vi "Autonomous Independent.vi"   [LabVIEW 2016]
doc: "This VI is called when autonomous begins, and will automatically be terminated when autonomous ends. You can carry out timed or sensor driven robot movement independently without needing to return to the caller."
uses:
  <vilib>/Rock Robotics/Network Tables/NT Read String.vi
  Robot Global Data.vi
panel:
  # "Be sure to right-click and choose Data Operations>>Make Current Value default if you want to save the array values with the VI"
types:
  T1 = typedef "WPI_MotorControlDeviceRef.ctl" = cluster{"DeviceStatus":errorcluster, "Type":T2, "PWM":cluster{"PWM Channel":T3, "DeadBand":T4}, "CAN":cluster{"Device Number":u8, "SetOutput VI Ref":variant, "GetOutput VI Ref":variant, "Enable VI Ref":variant, "Disable VI Ref":variant, "Data":variant}, "Invert":bool}
  T2 = typedef "WPI_MotorControlType.ctl" = enum16{"PWM", "CAN"}
  T3 = typedef "FPGA_DIOPWMChannel.ctl" = enum8{"PWM 0", "PWM 1", "PWM 2", "PWM 3", "PWM 4", "PWM 5", "PWM 6", "PWM 7", "PWM 8", "PWM 9", "PWM MXP 0", "PWM MXP 1", "PWM MXP 2", "PWM MXP 3", "PWM MXP 4", "PWM MXP 5", "PWM MXP 6", "PWM MXP 7", "PWM MXP 8", "PWM MXP 9", "Invalid"}
  T4 = typedef "WPI_PWMDeadband.ctl" = cluster{"Name":string, "maxPositivePwm":i32, "minPositivePwm":i32, "centerPwm":i32, "maxNegativePwm":i32, "minNegativePwm":i32, "angularRange":u16}
  T5 = typedef "WPI_CANTalonSRX_GlobalStatus.ctl" = cluster{"Applied Throttle":dbl, "Module Enabled":bool, "CAN Error":errorcluster, "Closed Loop Error":dbl, "Forward Limit Switch Closed":bool, "Reverse Limit Switch Closed":bool, "Sensor Position":dbl, "Sensor Velocity":dbl, "Current":dbl, "Sticky Fault - Over Temp":bool, "Sticky Fault - Under Voltage":bool, "Sticky Fault - Forward Limit":bool, "Sticky Fault - Reverse Limit":bool, "Sticky Fault - Forward Soft Limit":bool, "Sticky Fault - Reverse Soft Limit":bool, "Brake is Enabled":bool, "Encoder Position":dbl, "Encoder Velocity":dbl, "Encoder Index Count":dbl, "Encoder A Pin State":bool, "Encoder B Pin State":bool, "Encoder Index Pin State":bool, "Analog In":dbl, "Analog In Velocity":dbl, "Temperature (C)":dbl, "Battery Voltage":dbl, "Control 5 Is Supported":bool, "Current Profile Slot Select":dbl, "Pos Div 8":bool, "Vel Div 4":bool, "Pulse Width Position":i32, "Pulse Width Velocity":i32, "Pulse Width Rise To Rise (us)":i32, "Pulse Width Rise To Fall (us)":i32, "Mot Prof Active Is Under Run":bool, "Mot Prof Active Has Under Run":bool, "Mot Prof Active Is Last":bool, "Mot Prof Active Velocity Only":bool, "Mot Prof Active Is Valid":bool, "Mot Prof Buffer Is Full":bool, "Mot Prof Active Profile Slot Select":i32, "Mot Prof NextID":i32, "Mot Prof Count":i32, "Mot Prof Active Velocity":dbl, "Mot Prof Active Position":dbl, "Mot Prof Output Enable":i32}
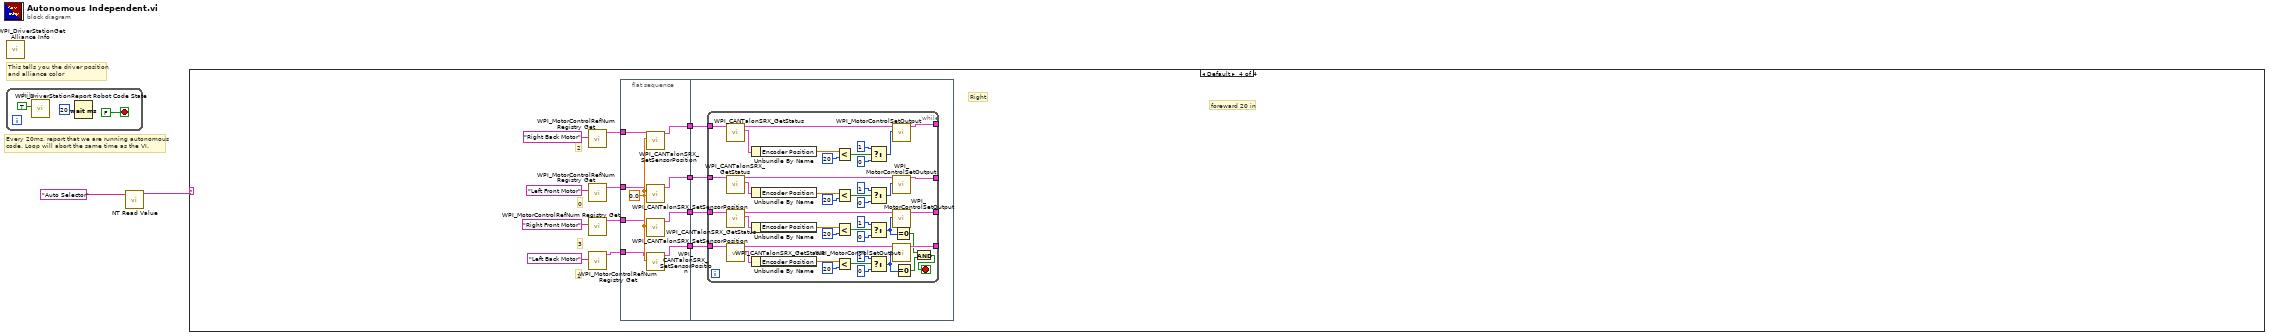
[diagram p0: block diagram]
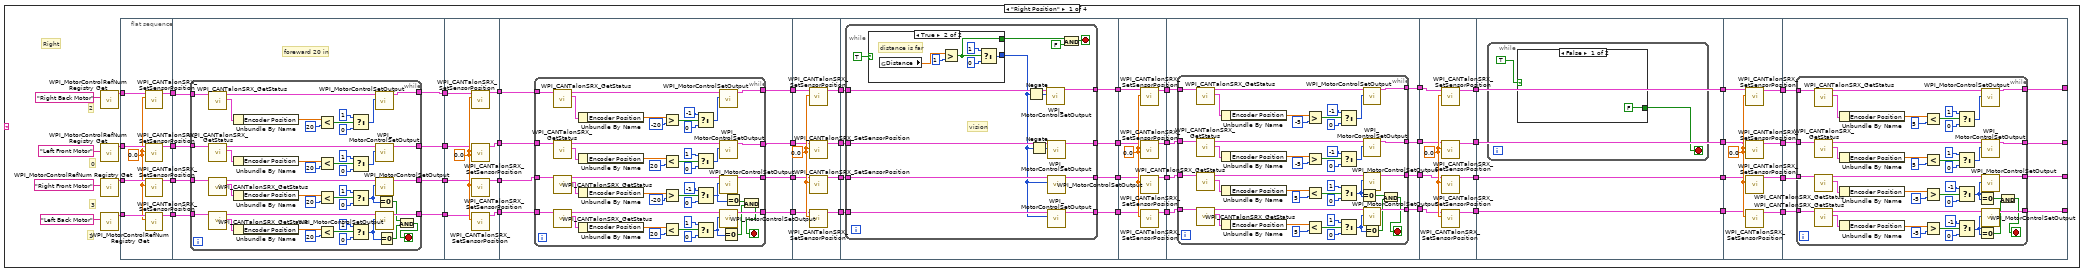
[diagram p2: hidden frame]
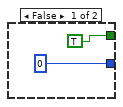
[diagram p3: hidden frame]
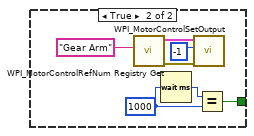
[diagram p4: hidden frame]
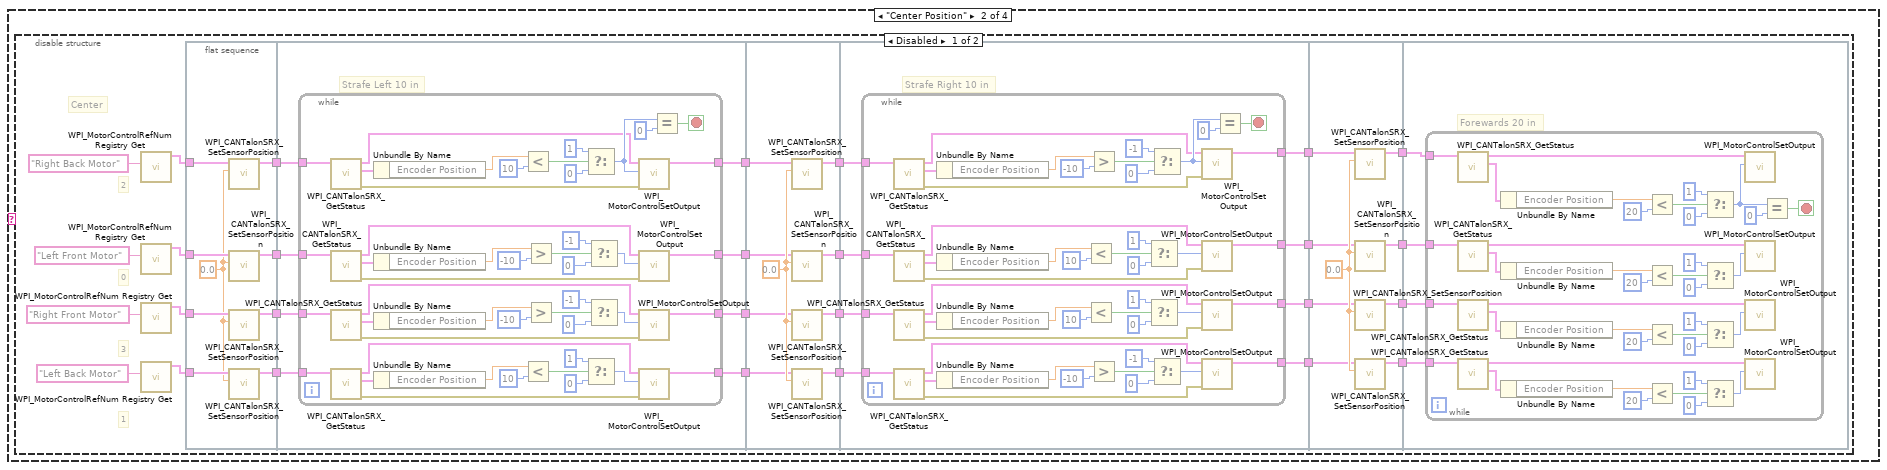
[diagram p5: hidden frame]
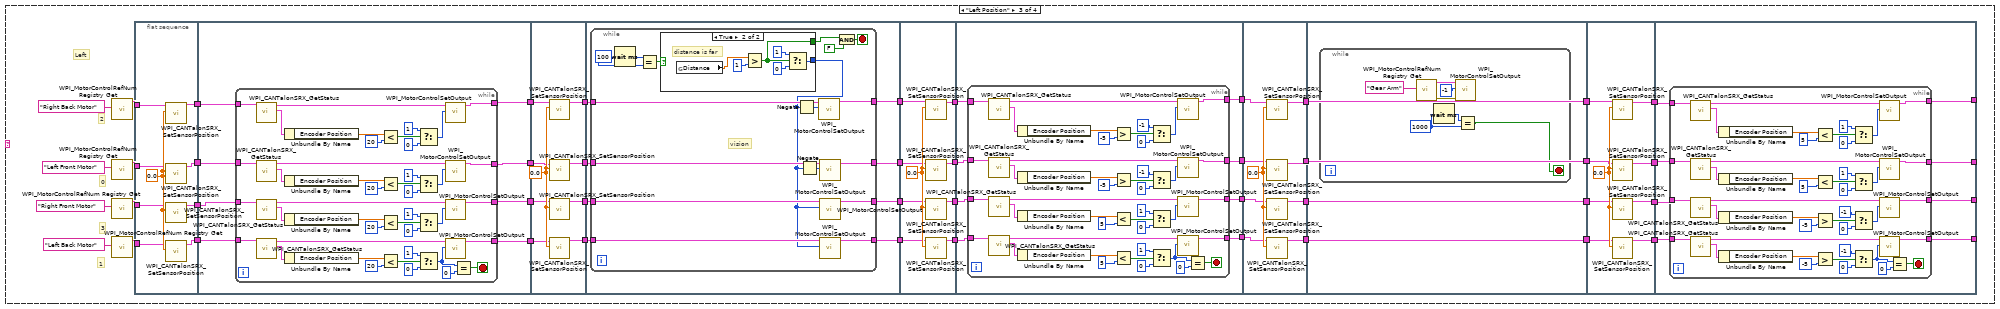
[diagram p7: hidden frame]
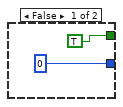
[diagram p8: hidden frame]
diagram:
  # "Every 20ms, report that we are running autonomous\ncode. Loop will abort the same time as the VI."
  # "This tells you the driver position\nand alliance color"
  n1 = call <vilib>:"WPI_DriverStationGet Alliance Info.vi"() -> ()  [unwired: 12 out]
  n2 = while {
    stop <- FALSE stop-if-true
    n3 = call <vilib>:"WPI_DriverStationReport Robot Code State.vi"("Autonomous"=TRUE) -> ()  [unwired: 10 in, 1 out]
    n4 = Wait (ms)(milliseconds to wait=u32 20) -> ()  [unwired: 1 out]
  }
  n5 = call-poly <vilib>:"NT Read Value.vi"("Name"="Auto Selector") -> ("String"=w1:string)  [unwired: 9 in, 1 out]
  n6 = case shown="Default" w1 {
    frame "Right Position" {
      # "Right"
      # "3"
      # "2"
      # "1"
      # "0"
      n7 = call <vilib>:"WPI_MotorControlRefNum Registry Get.vi"("refnum name"="Right Back Motor") -> ("MotorControlDevRef"=w42:T1)  [unwired: 9 in, 1 out]
      n8 = call <vilib>:"WPI_MotorControlRefNum Registry Get.vi"("refnum name"="Left Front Motor") -> ("MotorControlDevRef"=w43:T1)  [unwired: 9 in, 1 out]
      n9 = call <vilib>:"WPI_MotorControlRefNum Registry Get.vi"("refnum name"="Right Front Motor") -> ("MotorControlDevRef"=w44:T1)  [unwired: 9 in, 1 out]
      n10 = call <vilib>:"WPI_MotorControlRefNum Registry Get.vi"("refnum name"="Left Back Motor") -> ("MotorControlDevRef"=w45:T1)  [unwired: 9 in, 1 out]
      n11 = flat-sequence {
        tunnel: w45 -> [w65]
        tunnel: [w63] -> w57
        tunnel: w44 -> [w64]
        tunnel: w43 -> [w61]
        tunnel: [w59] -> w56
        tunnel: w42 -> [w60]
        tunnel: [w66] -> w55
        tunnel: [w62] -> w54
        tunnel: w57 -> [w71]
        tunnel: w56 -> [w73]
        tunnel: [w69] -> w53
        tunnel: [w68] -> w52
        tunnel: [w74] -> w51
        tunnel: w55 -> [w70]
        tunnel: w54 -> [w72]
        tunnel: [w67] -> w50
        tunnel: w53 -> [w122]
        tunnel: w52 -> [w123]
        tunnel: w51 -> [w125]
        tunnel: w50 -> [w124]
        tunnel: [w121] -> w37
        tunnel: [w120] -> w36
        tunnel: [w119] -> w35
        tunnel: [w118] -> w34
        tunnel: [w134] -> w41
        tunnel: [w133] -> w40
        tunnel: [w132] -> w39
        tunnel: [w131] -> w38
        tunnel: w37 -> [w130]
        tunnel: w36 -> [w129]
        tunnel: w35 -> [w128]
        tunnel: w34 -> [w127]
        tunnel: w41 -> [w185]
        tunnel: w40 -> [w184]
        tunnel: w39 -> [w183]
        tunnel: w38 -> [w182]
        tunnel: [w181] -> w33
        tunnel: [w180] -> w32
        tunnel: [w179] -> w31
        tunnel: [w178] -> w30
        tunnel: w33 -> [w194]
        tunnel: w32 -> [w193]
        tunnel: w31 -> [w192]
        tunnel: w30 -> [w191]
        tunnel: [w190] -> w29
        tunnel: [w189] -> w28
        tunnel: [w188] -> w27
        tunnel: [w187] -> w26
        tunnel: w29 -> [w225]
        tunnel: w28 -> [w224]
        tunnel: w27 -> [w223]
        tunnel: w26 -> [w222]
        tunnel: [w221] -> w25
        tunnel: [w220] -> w24
        tunnel: [w219] -> w23
        tunnel: [w218] -> w22
        tunnel: w25 -> [w231]
        tunnel: w24 -> [w232]
        tunnel: w23 -> [w233]
        tunnel: w22 -> [w234]
        tunnel: [w230] -> w21
        tunnel: [w229] -> w20
        tunnel: [w228] -> w19
        tunnel: [w227] -> w18
        tunnel: w21 -> [w285]
        tunnel: w20 -> [w283]
        tunnel: w19 -> [w281]
        tunnel: w18 -> [w279]
        tunnel: [w284] -> w17
        tunnel: [w282] -> w16
        tunnel: [w280] -> w15
        tunnel: [w278] -> w14
        tunnel: w17 -> [w290]
        tunnel: w16 -> [w289]
        tunnel: w15 -> [w288]
        tunnel: w14 -> [w287]
        tunnel: [w290] -> w13
        tunnel: [w289] -> w12
        tunnel: [w288] -> w11
        tunnel: [w287] -> w10
        tunnel: w13 -> [w308]
        tunnel: w12 -> [w307]
        tunnel: w11 -> [w306]
        tunnel: w10 -> [w305]
        tunnel: [w304] -> w9
        tunnel: [w303] -> w8
        tunnel: [w302] -> w7
        tunnel: [w301] -> w6
        tunnel: w9 -> [w314]
        tunnel: w8 -> [w315]
        tunnel: w7 -> [w316]
        tunnel: w6 -> [w317]
        tunnel: [w313] -> _
        tunnel: [w312] -> _
        tunnel: [w311] -> _
        tunnel: [w310] -> _
        frame #0 {
          w58 = 0.0
          n12 = call <vilib>:"WPI_CANTalonSRX_SetSensorPosition.vi"("New Sensor Position"=w58, "CAN Talon SRX Ref"=w60) -> ("CAN Talon SRX Ref"=w59:T1)  [unwired: 8 in, 1 out]
          n13 = call <vilib>:"WPI_CANTalonSRX_SetSensorPosition.vi"("New Sensor Position"=w58, "CAN Talon SRX Ref"=w61) -> ("CAN Talon SRX Ref"=w62:T1)  [unwired: 8 in, 1 out]
          n14 = call <vilib>:"WPI_CANTalonSRX_SetSensorPosition.vi"("New Sensor Position"=w58, "CAN Talon SRX Ref"=w64) -> ("CAN Talon SRX Ref"=w63:T1)  [unwired: 8 in, 1 out]
          n15 = call <vilib>:"WPI_CANTalonSRX_SetSensorPosition.vi"("New Sensor Position"=w58, "CAN Talon SRX Ref"=w65) -> ("CAN Talon SRX Ref"=w66:T1)  [unwired: 8 in, 1 out]
        }
        frame #1 {
          # "foreward 20 in"
          n16 = while {
            tunnel: w73 -> [w88]
            tunnel: w72 -> [w87]
            tunnel: w71 -> [w86]
            tunnel: w70 -> [w85]
            tunnel: [w83] -> w74
            tunnel: [w82] -> w69
            tunnel: [w81] -> w68
            tunnel: [w80] -> w67
            stop <- w75 stop-if-true
            n17 = call <vilib>:"WPI_CANTalonSRX_GetStatus.vi"("CAN Talon SRX Ref"=w88) -> ("Talon SRX Status"=w97:T5, "CAN Talon SRX Ref"=w96:T1)  [unwired: 8 in, 1 out]
            n18 = call <vilib>:"WPI_CANTalonSRX_GetStatus.vi"("CAN Talon SRX Ref"=w87) -> ("Talon SRX Status"=w100:T5, "CAN Talon SRX Ref"=w93:T1)  [unwired: 8 in, 1 out]
            n19 = call <vilib>:"WPI_CANTalonSRX_GetStatus.vi"("CAN Talon SRX Ref"=w86) -> ("Talon SRX Status"=w99:T5, "CAN Talon SRX Ref"=w95:T1)  [unwired: 8 in, 1 out]
            n20 = call <vilib>:"WPI_CANTalonSRX_GetStatus.vi"("CAN Talon SRX Ref"=w85) -> ("Talon SRX Status"=w98:T5, "CAN Talon SRX Ref"=w94:T1)  [unwired: 8 in, 1 out]
            n21 = Unbundle By Name(w97) -> ("Encoder Position"=w89:dbl)
            n22 = Unbundle By Name(w100) -> ("Encoder Position"=w92:dbl)
            n23 = Unbundle By Name(w99) -> ("Encoder Position"=w90:dbl)
            n24 = Unbundle By Name(w98) -> ("Encoder Position"=w91:dbl)
            n25 = Less?(x=w89, y=20) -> (x < y?=w103:bool)
            n26 = Less?(x=w92, y=20) -> (x < y?=w111:bool)
            n27 = Less?(x=w90, y=20) -> (x < y?=w109:bool)
            n28 = Less?(x=w91, y=20) -> (x < y?=w110:bool)
            n29 = Select(t=1, s=w103, f=0) -> (s? t:f=w101:i32)
            n30 = Select(t=1, s=w111, f=0) -> (s? t:f=w112:i32)
            n31 = Select(t=1, s=w109, f=0) -> (s? t:f=w79:i32)
            n32 = Select(t=1, s=w110, f=0) -> (s? t:f=w78:i32)
            n33 = call <vilib>:"WPI_MotorControlSetOutput.vi"("Output"=w101, "MotorControlDevRef"=w96) -> ("MotorControlDevRef"=w83:T1)  [unwired: 7 in, 2 out]
            n34 = call <vilib>:"WPI_MotorControlSetOutput.vi"("Output"=w112, "MotorControlDevRef"=w93) -> ("MotorControlDevRef"=w80:T1)  [unwired: 7 in, 2 out]
            n35 = call <vilib>:"WPI_MotorControlSetOutput.vi"("Output"=w79, "MotorControlDevRef"=w95) -> ("MotorControlDevRef"=w81:T1)  [unwired: 7 in, 2 out]
            n36 = call <vilib>:"WPI_MotorControlSetOutput.vi"("Output"=w78, "MotorControlDevRef"=w94) -> ("MotorControlDevRef"=w82:T1)  [unwired: 7 in, 2 out]
            n37 = Equal To 0?(x=w79) -> (x = 0?=w77:bool)
            n38 = Equal To 0?(x=w78) -> (x = 0?=w76:bool)
            n39 = And(x=w77, y=w76) -> (x .and. y?=w75:bool)
          }
        }
        frame #2 {
          w126 = 0.0
          n40 = call <vilib>:"WPI_CANTalonSRX_SetSensorPosition.vi"("New Sensor Position"=w126, "CAN Talon SRX Ref"=w125) -> ("CAN Talon SRX Ref"=w118:T1)  [unwired: 8 in, 1 out]
          n41 = call <vilib>:"WPI_CANTalonSRX_SetSensorPosition.vi"("New Sensor Position"=w126, "CAN Talon SRX Ref"=w124) -> ("CAN Talon SRX Ref"=w119:T1)  [unwired: 8 in, 1 out]
          n42 = call <vilib>:"WPI_CANTalonSRX_SetSensorPosition.vi"("New Sensor Position"=w126, "CAN Talon SRX Ref"=w123) -> ("CAN Talon SRX Ref"=w120:T1)  [unwired: 8 in, 1 out]
          n43 = call <vilib>:"WPI_CANTalonSRX_SetSensorPosition.vi"("New Sensor Position"=w126, "CAN Talon SRX Ref"=w122) -> ("CAN Talon SRX Ref"=w121:T1)  [unwired: 8 in, 1 out]
        }
        frame #3 {
          n44 = while {
            tunnel: w127 -> [w148]
            tunnel: w128 -> [w147]
            tunnel: w129 -> [w146]
            tunnel: w130 -> [w145]
            tunnel: [w143] -> w131
            tunnel: [w142] -> w134
            tunnel: [w141] -> w133
            tunnel: [w140] -> w132
            stop <- w135 stop-if-true
            n45 = call <vilib>:"WPI_CANTalonSRX_GetStatus.vi"("CAN Talon SRX Ref"=w148) -> ("Talon SRX Status"=w157:T5, "CAN Talon SRX Ref"=w156:T1)  [unwired: 8 in, 1 out]
            n46 = call <vilib>:"WPI_CANTalonSRX_GetStatus.vi"("CAN Talon SRX Ref"=w147) -> ("Talon SRX Status"=w160:T5, "CAN Talon SRX Ref"=w153:T1)  [unwired: 8 in, 1 out]
            n47 = call <vilib>:"WPI_CANTalonSRX_GetStatus.vi"("CAN Talon SRX Ref"=w146) -> ("Talon SRX Status"=w159:T5, "CAN Talon SRX Ref"=w155:T1)  [unwired: 8 in, 1 out]
            n48 = call <vilib>:"WPI_CANTalonSRX_GetStatus.vi"("CAN Talon SRX Ref"=w145) -> ("Talon SRX Status"=w158:T5, "CAN Talon SRX Ref"=w154:T1)  [unwired: 8 in, 1 out]
            n49 = Unbundle By Name(w157) -> ("Encoder Position"=w149:dbl)
            n50 = Unbundle By Name(w160) -> ("Encoder Position"=w152:dbl)
            n51 = Unbundle By Name(w159) -> ("Encoder Position"=w150:dbl)
            n52 = Unbundle By Name(w158) -> ("Encoder Position"=w151:dbl)
            n53 = Greater?(x=w149, y=-20) -> (0:w163:bool)
            n54 = Less?(x=w152, y=20) -> (x < y?=w171:bool)
            n55 = Greater?(x=w150, y=-20) -> (0:w169:bool)
            n56 = Less?(x=w151, y=20) -> (x < y?=w170:bool)
            n57 = Select(t=-1, s=w163, f=0) -> (s? t:f=w161:i32)
            n58 = Select(t=1, s=w171, f=0) -> (s? t:f=w172:i32)
            n59 = Select(t=-1, s=w169, f=0) -> (s? t:f=w138:i32)
            n60 = Select(t=1, s=w170, f=0) -> (s? t:f=w139:i32)
            n61 = call <vilib>:"WPI_MotorControlSetOutput.vi"("Output"=w161, "MotorControlDevRef"=w156) -> ("MotorControlDevRef"=w143:T1)  [unwired: 7 in, 2 out]
            n62 = call <vilib>:"WPI_MotorControlSetOutput.vi"("Output"=w172, "MotorControlDevRef"=w153) -> ("MotorControlDevRef"=w140:T1)  [unwired: 7 in, 2 out]
            n63 = call <vilib>:"WPI_MotorControlSetOutput.vi"("Output"=w138, "MotorControlDevRef"=w155) -> ("MotorControlDevRef"=w141:T1)  [unwired: 7 in, 2 out]
            n64 = call <vilib>:"WPI_MotorControlSetOutput.vi"("Output"=w139, "MotorControlDevRef"=w154) -> ("MotorControlDevRef"=w142:T1)  [unwired: 7 in, 2 out]
            n65 = Equal To 0?(x=w139) -> (x = 0?=w136:bool)
            n66 = Equal To 0?(x=w138) -> (x = 0?=w137:bool)
            n67 = And(x=w137, y=w136) -> (x .and. y?=w135:bool)
          }
        }
        frame #4 {
          w186 = 0.0
          n68 = call <vilib>:"WPI_CANTalonSRX_SetSensorPosition.vi"("New Sensor Position"=w186, "CAN Talon SRX Ref"=w182) -> ("CAN Talon SRX Ref"=w181:T1)  [unwired: 8 in, 1 out]
          n69 = call <vilib>:"WPI_CANTalonSRX_SetSensorPosition.vi"("New Sensor Position"=w186, "CAN Talon SRX Ref"=w183) -> ("CAN Talon SRX Ref"=w180:T1)  [unwired: 8 in, 1 out]
          n70 = call <vilib>:"WPI_CANTalonSRX_SetSensorPosition.vi"("New Sensor Position"=w186, "CAN Talon SRX Ref"=w184) -> ("CAN Talon SRX Ref"=w179:T1)  [unwired: 8 in, 1 out]
          n71 = call <vilib>:"WPI_CANTalonSRX_SetSensorPosition.vi"("New Sensor Position"=w186, "CAN Talon SRX Ref"=w185) -> ("CAN Talon SRX Ref"=w178:T1)  [unwired: 8 in, 1 out]
        }
        frame #5 {
          n72 = while {
            tunnel: w194 -> [w209]
            tunnel: w193 -> [w208]
            tunnel: w192 -> [w207]
            tunnel: w191 -> [w206]
            tunnel: [w205] -> w190
            tunnel: [w204] -> w189
            tunnel: [w203] -> w188
            tunnel: [w202] -> w187
            stop <- w198 stop-if-true
            # "vision"
            n73 = case shown="True" TRUE {
              tunnel: [0 w214] -> w201
              tunnel: [TRUE w213] -> w197
              frame False {
              }
              frame True {
                # "distance is far"
                n74 = global read "Robot Global Data.vi" "Distance"() -> (w212:dbl)
                n75 = Greater?(x=w212, y=1) -> (0:w213:bool)
                n76 = Select(t=1, s=w213, f=0) -> (s? t:f=w214:i32)
              }
            }
            n77 = Negate(x=w201) -> (-x=w200:i32)
            n78 = Negate(x=w201) -> (-x=w199:i32)
            n79 = call <vilib>:"WPI_MotorControlSetOutput.vi"("Output"=w200, "MotorControlDevRef"=w209) -> ("MotorControlDevRef"=w205:T1)  [unwired: 7 in, 2 out]
            n80 = call <vilib>:"WPI_MotorControlSetOutput.vi"("Output"=w199, "MotorControlDevRef"=w208) -> ("MotorControlDevRef"=w204:T1)  [unwired: 7 in, 2 out]
            n81 = call <vilib>:"WPI_MotorControlSetOutput.vi"("Output"=w201, "MotorControlDevRef"=w207) -> ("MotorControlDevRef"=w203:T1)  [unwired: 7 in, 2 out]
            n82 = call <vilib>:"WPI_MotorControlSetOutput.vi"("Output"=w201, "MotorControlDevRef"=w206) -> ("MotorControlDevRef"=w202:T1)  [unwired: 7 in, 2 out]
            n83 = And(x=w197, y=FALSE) -> (x .and. y?=w198:bool)
          }
        }
        frame #6 {
          w226 = 0.0
          n84 = call <vilib>:"WPI_CANTalonSRX_SetSensorPosition.vi"("New Sensor Position"=w226, "CAN Talon SRX Ref"=w225) -> ("CAN Talon SRX Ref"=w218:T1)  [unwired: 8 in, 1 out]
          n85 = call <vilib>:"WPI_CANTalonSRX_SetSensorPosition.vi"("New Sensor Position"=w226, "CAN Talon SRX Ref"=w224) -> ("CAN Talon SRX Ref"=w219:T1)  [unwired: 8 in, 1 out]
          n86 = call <vilib>:"WPI_CANTalonSRX_SetSensorPosition.vi"("New Sensor Position"=w226, "CAN Talon SRX Ref"=w223) -> ("CAN Talon SRX Ref"=w220:T1)  [unwired: 8 in, 1 out]
          n87 = call <vilib>:"WPI_CANTalonSRX_SetSensorPosition.vi"("New Sensor Position"=w226, "CAN Talon SRX Ref"=w222) -> ("CAN Talon SRX Ref"=w221:T1)  [unwired: 8 in, 1 out]
        }
        frame #7 {
          n88 = while {
            tunnel: w234 -> [w248]
            tunnel: w233 -> [w247]
            tunnel: w232 -> [w246]
            tunnel: w231 -> [w245]
            tunnel: [w243] -> w230
            tunnel: [w242] -> w227
            tunnel: [w241] -> w228
            tunnel: [w240] -> w229
            stop <- w235 stop-if-true
            n89 = call <vilib>:"WPI_CANTalonSRX_GetStatus.vi"("CAN Talon SRX Ref"=w248) -> ("Talon SRX Status"=w257:T5, "CAN Talon SRX Ref"=w256:T1)  [unwired: 8 in, 1 out]
            n90 = call <vilib>:"WPI_CANTalonSRX_GetStatus.vi"("CAN Talon SRX Ref"=w247) -> ("Talon SRX Status"=w260:T5, "CAN Talon SRX Ref"=w253:T1)  [unwired: 8 in, 1 out]
            n91 = call <vilib>:"WPI_CANTalonSRX_GetStatus.vi"("CAN Talon SRX Ref"=w246) -> ("Talon SRX Status"=w259:T5, "CAN Talon SRX Ref"=w255:T1)  [unwired: 8 in, 1 out]
            n92 = call <vilib>:"WPI_CANTalonSRX_GetStatus.vi"("CAN Talon SRX Ref"=w245) -> ("Talon SRX Status"=w258:T5, "CAN Talon SRX Ref"=w254:T1)  [unwired: 8 in, 1 out]
            n93 = Unbundle By Name(w257) -> ("Encoder Position"=w249:dbl)
            n94 = Unbundle By Name(w260) -> ("Encoder Position"=w252:dbl)
            n95 = Unbundle By Name(w259) -> ("Encoder Position"=w250:dbl)
            n96 = Unbundle By Name(w258) -> ("Encoder Position"=w251:dbl)
            n97 = Greater?(x=w249, y=-5) -> (0:w263:bool)
            n98 = Greater?(x=w252, y=-5) -> (0:w271:bool)
            n99 = Less?(x=w250, y=5) -> (x < y?=w269:bool)
            n100 = Less?(x=w251, y=5) -> (x < y?=w270:bool)
            n101 = Select(t=-1, s=w263, f=0) -> (s? t:f=w261:i32)
            n102 = Select(t=-1, s=w271, f=0) -> (s? t:f=w272:i32)
            n103 = Select(t=1, s=w269, f=0) -> (s? t:f=w239:i32)
            n104 = Select(t=1, s=w270, f=0) -> (s? t:f=w237:i32)
            n105 = Equal To 0?(x=w239) -> (x = 0?=w238:bool)
            n106 = call <vilib>:"WPI_MotorControlSetOutput.vi"("Output"=w261, "MotorControlDevRef"=w256) -> ("MotorControlDevRef"=w243:T1)  [unwired: 7 in, 2 out]
            n107 = call <vilib>:"WPI_MotorControlSetOutput.vi"("Output"=w272, "MotorControlDevRef"=w253) -> ("MotorControlDevRef"=w240:T1)  [unwired: 7 in, 2 out]
            n108 = call <vilib>:"WPI_MotorControlSetOutput.vi"("Output"=w239, "MotorControlDevRef"=w255) -> ("MotorControlDevRef"=w241:T1)  [unwired: 7 in, 2 out]
            n109 = call <vilib>:"WPI_MotorControlSetOutput.vi"("Output"=w237, "MotorControlDevRef"=w254) -> ("MotorControlDevRef"=w242:T1)  [unwired: 7 in, 2 out]
            n110 = Equal To 0?(x=w237) -> (x = 0?=w236:bool)
            n111 = And(x=w238, y=w236) -> (x .and. y?=w235:bool)
          }
        }
        frame #8 {
          w286 = 0.0
          n112 = call <vilib>:"WPI_CANTalonSRX_SetSensorPosition.vi"("New Sensor Position"=w286, "CAN Talon SRX Ref"=w285) -> ("CAN Talon SRX Ref"=w284:T1)  [unwired: 8 in, 1 out]
          n113 = call <vilib>:"WPI_CANTalonSRX_SetSensorPosition.vi"("New Sensor Position"=w286, "CAN Talon SRX Ref"=w283) -> ("CAN Talon SRX Ref"=w282:T1)  [unwired: 8 in, 1 out]
          n114 = call <vilib>:"WPI_CANTalonSRX_SetSensorPosition.vi"("New Sensor Position"=w286, "CAN Talon SRX Ref"=w281) -> ("CAN Talon SRX Ref"=w280:T1)  [unwired: 8 in, 1 out]
          n115 = call <vilib>:"WPI_CANTalonSRX_SetSensorPosition.vi"("New Sensor Position"=w286, "CAN Talon SRX Ref"=w279) -> ("CAN Talon SRX Ref"=w278:T1)  [unwired: 8 in, 1 out]
        }
        frame #9 {
          n116 = while {
            stop <- w291 stop-if-true
            n117 = case shown="False" TRUE {
              tunnel: [FALSE w294] -> w291
              frame False {
              }
              frame True {
                w295 = 1000
                n118 = call <vilib>:"WPI_MotorControlRefNum Registry Get.vi"("refnum name"="Gear Arm") -> ("error out"=w300:errorcluster, "MotorControlDevRef"=w299:T1)  [unwired: 9 in]
                n119 = Wait (ms)(milliseconds to wait=w295) -> (millisecond timer value=w296:u32)
                n120 = call <vilib>:"WPI_MotorControlSetOutput.vi"("error in (no error)"=w300, "Output"=-1, "MotorControlDevRef"=w299) -> ()  [unwired: 6 in, 3 out]
                n121 = Equal?(x=w296, y=w295) -> (x = y?=w294:bool)
              }
            }
          }
        }
        frame #10 {
          w309 = 0.0
          n122 = call <vilib>:"WPI_CANTalonSRX_SetSensorPosition.vi"("New Sensor Position"=w309, "CAN Talon SRX Ref"=w308) -> ("CAN Talon SRX Ref"=w301:T1)  [unwired: 8 in, 1 out]
          n123 = call <vilib>:"WPI_CANTalonSRX_SetSensorPosition.vi"("New Sensor Position"=w309, "CAN Talon SRX Ref"=w307) -> ("CAN Talon SRX Ref"=w302:T1)  [unwired: 8 in, 1 out]
          n124 = call <vilib>:"WPI_CANTalonSRX_SetSensorPosition.vi"("New Sensor Position"=w309, "CAN Talon SRX Ref"=w306) -> ("CAN Talon SRX Ref"=w303:T1)  [unwired: 8 in, 1 out]
          n125 = call <vilib>:"WPI_CANTalonSRX_SetSensorPosition.vi"("New Sensor Position"=w309, "CAN Talon SRX Ref"=w305) -> ("CAN Talon SRX Ref"=w304:T1)  [unwired: 8 in, 1 out]
        }
        frame #11 {
          n126 = while {
            tunnel: w317 -> [w331]
            tunnel: w316 -> [w330]
            tunnel: w315 -> [w329]
            tunnel: w314 -> [w328]
            tunnel: [w326] -> w313
            tunnel: [w325] -> w310
            tunnel: [w324] -> w311
            tunnel: [w323] -> w312
            stop <- w318 stop-if-true
            n127 = call <vilib>:"WPI_CANTalonSRX_GetStatus.vi"("CAN Talon SRX Ref"=w331) -> ("Talon SRX Status"=w340:T5, "CAN Talon SRX Ref"=w339:T1)  [unwired: 8 in, 1 out]
            n128 = call <vilib>:"WPI_CANTalonSRX_GetStatus.vi"("CAN Talon SRX Ref"=w330) -> ("Talon SRX Status"=w343:T5, "CAN Talon SRX Ref"=w336:T1)  [unwired: 8 in, 1 out]
            n129 = call <vilib>:"WPI_CANTalonSRX_GetStatus.vi"("CAN Talon SRX Ref"=w329) -> ("Talon SRX Status"=w342:T5, "CAN Talon SRX Ref"=w338:T1)  [unwired: 8 in, 1 out]
            n130 = call <vilib>:"WPI_CANTalonSRX_GetStatus.vi"("CAN Talon SRX Ref"=w328) -> ("Talon SRX Status"=w341:T5, "CAN Talon SRX Ref"=w337:T1)  [unwired: 8 in, 1 out]
            n131 = Unbundle By Name(w340) -> ("Encoder Position"=w332:dbl)
            n132 = Unbundle By Name(w343) -> ("Encoder Position"=w335:dbl)
            n133 = Unbundle By Name(w342) -> ("Encoder Position"=w333:dbl)
            n134 = Unbundle By Name(w341) -> ("Encoder Position"=w334:dbl)
            n135 = Less?(x=w332, y=5) -> (x < y?=w346:bool)
            n136 = Less?(x=w335, y=5) -> (x < y?=w354:bool)
            n137 = Greater?(x=w333, y=-5) -> (0:w352:bool)
            n138 = Greater?(x=w334, y=-5) -> (0:w353:bool)
            n139 = Select(t=1, s=w346, f=0) -> (s? t:f=w344:i32)
            n140 = Select(t=1, s=w354, f=0) -> (s? t:f=w355:i32)
            n141 = Select(t=-1, s=w352, f=0) -> (s? t:f=w321:i32)
            n142 = Select(t=-1, s=w353, f=0) -> (s? t:f=w320:i32)
            n143 = Equal To 0?(x=w321) -> (x = 0?=w322:bool)
            n144 = Equal To 0?(x=w320) -> (x = 0?=w319:bool)
            n145 = call <vilib>:"WPI_MotorControlSetOutput.vi"("Output"=w344, "MotorControlDevRef"=w339) -> ("MotorControlDevRef"=w326:T1)  [unwired: 7 in, 2 out]
            n146 = call <vilib>:"WPI_MotorControlSetOutput.vi"("Output"=w355, "MotorControlDevRef"=w336) -> ("MotorControlDevRef"=w323:T1)  [unwired: 7 in, 2 out]
            n147 = call <vilib>:"WPI_MotorControlSetOutput.vi"("Output"=w321, "MotorControlDevRef"=w338) -> ("MotorControlDevRef"=w324:T1)  [unwired: 7 in, 2 out]
            n148 = call <vilib>:"WPI_MotorControlSetOutput.vi"("Output"=w320, "MotorControlDevRef"=w337) -> ("MotorControlDevRef"=w325:T1)  [unwired: 7 in, 2 out]
            n149 = And(x=w322, y=w319) -> (x .and. y?=w318:bool)
          }
        }
      }
    }
    frame "Center Position" {
      n150 = disable-structure shown="Disabled" {
        frame Disabled {
          # "Center"
          # "3"
          # "2"
          # "1"
          # "0"
          n151 = call <vilib>:"WPI_MotorControlRefNum Registry Get.vi"("refnum name"="Right Back Motor") -> ("MotorControlDevRef"=w361:T1)  [unwired: 9 in, 1 out]
          n152 = call <vilib>:"WPI_MotorControlRefNum Registry Get.vi"("refnum name"="Left Front Motor") -> ("MotorControlDevRef"=w362:T1)  [unwired: 9 in, 1 out]
          n153 = call <vilib>:"WPI_MotorControlRefNum Registry Get.vi"("refnum name"="Right Front Motor") -> ("MotorControlDevRef"=w363:T1)  [unwired: 9 in, 1 out]
          n154 = call <vilib>:"WPI_MotorControlRefNum Registry Get.vi"("refnum name"="Left Back Motor") -> ("MotorControlDevRef"=w364:T1)  [unwired: 9 in, 1 out]
          n155 = flat-sequence {
            tunnel: w364 -> [w396]
            tunnel: [w394] -> w388
            tunnel: w363 -> [w395]
            tunnel: w362 -> [w392]
            tunnel: [w390] -> w387
            tunnel: w361 -> [w391]
            tunnel: [w397] -> w386
            tunnel: [w393] -> w385
            tunnel: w388 -> [w404]
            tunnel: w387 -> [w402]
            tunnel: [w401] -> w384
            tunnel: [w400] -> w383
            tunnel: [w399] -> w382
            tunnel: [w398] -> w381
            tunnel: w386 -> [w405]
            tunnel: w385 -> [w403]
            tunnel: [w452] -> w380
            tunnel: w384 -> [w453]
            tunnel: w383 -> [w454]
            tunnel: [w456] -> w379
            tunnel: w382 -> [w457]
            tunnel: w381 -> [w458]
            tunnel: [w459] -> w378
            tunnel: [w455] -> w377
            tunnel: w380 -> [w468]
            tunnel: w379 -> [w466]
            tunnel: [w464] -> w376
            tunnel: [w463] -> w375
            tunnel: [w462] -> w374
            tunnel: [w461] -> w373
            tunnel: w378 -> [w465]
            tunnel: w377 -> [w467]
            tunnel: [w521] -> w372
            tunnel: w376 -> [w522]
            tunnel: w375 -> [w515]
            tunnel: [w520] -> w371
            tunnel: w374 -> [w516]
            tunnel: w373 -> [w517]
            tunnel: [w519] -> w370
            tunnel: [w518] -> w369
            tunnel: w372 -> [w527]
            tunnel: w371 -> [w526]
            tunnel: w370 -> [w525]
            tunnel: w369 -> [w524]
            frame #0 {
              w389 = 0.0
              n156 = call <vilib>:"WPI_CANTalonSRX_SetSensorPosition.vi"("New Sensor Position"=w389, "CAN Talon SRX Ref"=w391) -> ("CAN Talon SRX Ref"=w390:T1)  [unwired: 8 in, 1 out]
              n157 = call <vilib>:"WPI_CANTalonSRX_SetSensorPosition.vi"("New Sensor Position"=w389, "CAN Talon SRX Ref"=w392) -> ("CAN Talon SRX Ref"=w393:T1)  [unwired: 8 in, 1 out]
              n158 = call <vilib>:"WPI_CANTalonSRX_SetSensorPosition.vi"("New Sensor Position"=w389, "CAN Talon SRX Ref"=w395) -> ("CAN Talon SRX Ref"=w394:T1)  [unwired: 8 in, 1 out]
              n159 = call <vilib>:"WPI_CANTalonSRX_SetSensorPosition.vi"("New Sensor Position"=w389, "CAN Talon SRX Ref"=w396) -> ("CAN Talon SRX Ref"=w397:T1)  [unwired: 8 in, 1 out]
            }
            frame #1 {
              # "Strafe Left 10 in"
              n160 = while {
                tunnel: w405 -> [w414]
                tunnel: w404 -> [w413]
                tunnel: w403 -> [w412]
                tunnel: w402 -> [w411]
                tunnel: [w409] -> w401
                tunnel: [w408] -> w400
                tunnel: [w407] -> w399
                tunnel: [w406] -> w398
                stop <- w410 stop-if-true
                n161 = call <vilib>:"WPI_CANTalonSRX_GetStatus.vi"("CAN Talon SRX Ref"=w411) -> ("error out"=w422:errorcluster, "Talon SRX Status"=w415:T5, "CAN Talon SRX Ref"=w423:T1)  [unwired: 8 in]
                n162 = call <vilib>:"WPI_CANTalonSRX_GetStatus.vi"("CAN Talon SRX Ref"=w412) -> ("error out"=w418:errorcluster, "Talon SRX Status"=w417:T5, "CAN Talon SRX Ref"=w419:T1)  [unwired: 8 in]
                n163 = call <vilib>:"WPI_CANTalonSRX_GetStatus.vi"("CAN Talon SRX Ref"=w413) -> ("error out"=w420:errorcluster, "Talon SRX Status"=w416:T5, "CAN Talon SRX Ref"=w421:T1)  [unwired: 8 in]
                n164 = call <vilib>:"WPI_CANTalonSRX_GetStatus.vi"("CAN Talon SRX Ref"=w414) -> ("error out"=w426:errorcluster, "Talon SRX Status"=w425:T5, "CAN Talon SRX Ref"=w427:T1)  [unwired: 8 in]
                n165 = Unbundle By Name(w415) -> ("Encoder Position"=w449:dbl)
                n166 = Unbundle By Name(w417) -> ("Encoder Position"=w451:dbl)
                n167 = Unbundle By Name(w416) -> ("Encoder Position"=w450:dbl)
                n168 = Unbundle By Name(w425) -> ("Encoder Position"=w424:dbl)
                n169 = Less?(x=w449, y=10) -> (x < y?=w435:bool)
                n170 = Less?(x=w424, y=10) -> (x < y?=w429:bool)
                n171 = Greater?(x=w451, y=-10) -> (0:w437:bool)
                n172 = Greater?(x=w450, y=-10) -> (0:w439:bool)
                n173 = Select(t=1, s=w435, f=0) -> (s? t:f=w433:i32)
                n174 = Select(t=1, s=w429, f=0) -> (s? t:f=w430:i32)
                n175 = Select(t=-1, s=w437, f=0) -> (s? t:f=w441:i32)
                n176 = Select(t=-1, s=w439, f=0) -> (s? t:f=w442:i32)
                n177 = call <vilib>:"WPI_MotorControlSetOutput.vi"("error in (no error)"=w422, "Output"=w433, "MotorControlDevRef"=w423) -> ("MotorControlDevRef"=w406:T1)  [unwired: 6 in, 2 out]
                n178 = call <vilib>:"WPI_MotorControlSetOutput.vi"("error in (no error)"=w418, "Output"=w441, "MotorControlDevRef"=w419) -> ("MotorControlDevRef"=w407:T1)  [unwired: 6 in, 2 out]
                n179 = call <vilib>:"WPI_MotorControlSetOutput.vi"("error in (no error)"=w420, "Output"=w442, "MotorControlDevRef"=w421) -> ("MotorControlDevRef"=w408:T1)  [unwired: 6 in, 2 out]
                n180 = call <vilib>:"WPI_MotorControlSetOutput.vi"("error in (no error)"=w426, "Output"=w430, "MotorControlDevRef"=w427) -> ("MotorControlDevRef"=w409:T1)  [unwired: 6 in, 2 out]
                n181 = Equal?(x=w433, y=0) -> (x = y?=w410:bool)
              }
            }
            frame #2 {
              w460 = 0.0
              n182 = call <vilib>:"WPI_CANTalonSRX_SetSensorPosition.vi"("New Sensor Position"=w460, "CAN Talon SRX Ref"=w458) -> ("CAN Talon SRX Ref"=w459:T1)  [unwired: 8 in, 1 out]
              n183 = call <vilib>:"WPI_CANTalonSRX_SetSensorPosition.vi"("New Sensor Position"=w460, "CAN Talon SRX Ref"=w457) -> ("CAN Talon SRX Ref"=w456:T1)  [unwired: 8 in, 1 out]
              n184 = call <vilib>:"WPI_CANTalonSRX_SetSensorPosition.vi"("New Sensor Position"=w460, "CAN Talon SRX Ref"=w454) -> ("CAN Talon SRX Ref"=w455:T1)  [unwired: 8 in, 1 out]
              n185 = call <vilib>:"WPI_CANTalonSRX_SetSensorPosition.vi"("New Sensor Position"=w460, "CAN Talon SRX Ref"=w453) -> ("CAN Talon SRX Ref"=w452:T1)  [unwired: 8 in, 1 out]
            }
            frame #3 {
              # "Strafe Right 10 in"
              n186 = while {
                tunnel: w468 -> [w477]
                tunnel: w467 -> [w476]
                tunnel: w465 -> [w475]
                tunnel: w466 -> [w473]
                tunnel: [w472] -> w464
                tunnel: [w471] -> w463
                tunnel: [w470] -> w462
                tunnel: [w469] -> w461
                stop <- w474 stop-if-true
                n187 = call <vilib>:"WPI_CANTalonSRX_GetStatus.vi"("CAN Talon SRX Ref"=w475) -> ("error out"=w485:errorcluster, "Talon SRX Status"=w478:T5, "CAN Talon SRX Ref"=w486:T1)  [unwired: 8 in]
                n188 = call <vilib>:"WPI_CANTalonSRX_GetStatus.vi"("CAN Talon SRX Ref"=w473) -> ("error out"=w481:errorcluster, "Talon SRX Status"=w480:T5, "CAN Talon SRX Ref"=w482:T1)  [unwired: 8 in]
                n189 = call <vilib>:"WPI_CANTalonSRX_GetStatus.vi"("CAN Talon SRX Ref"=w476) -> ("error out"=w483:errorcluster, "Talon SRX Status"=w479:T5, "CAN Talon SRX Ref"=w484:T1)  [unwired: 8 in]
                n190 = call <vilib>:"WPI_CANTalonSRX_GetStatus.vi"("CAN Talon SRX Ref"=w477) -> ("error out"=w489:errorcluster, "Talon SRX Status"=w488:T5, "CAN Talon SRX Ref"=w490:T1)  [unwired: 8 in]
                n191 = Unbundle By Name(w478) -> ("Encoder Position"=w512:dbl)
                n192 = Unbundle By Name(w480) -> ("Encoder Position"=w514:dbl)
                n193 = Unbundle By Name(w479) -> ("Encoder Position"=w513:dbl)
                n194 = Unbundle By Name(w488) -> ("Encoder Position"=w487:dbl)
                n195 = Less?(x=w514, y=10) -> (x < y?=w500:bool)
                n196 = Less?(x=w513, y=10) -> (x < y?=w502:bool)
                n197 = Greater?(x=w512, y=-10) -> (0:w498:bool)
                n198 = Greater?(x=w487, y=-10) -> (0:w492:bool)
                n199 = Select(t=1, s=w500, f=0) -> (s? t:f=w504:i32)
                n200 = Select(t=1, s=w502, f=0) -> (s? t:f=w505:i32)
                n201 = Select(t=-1, s=w498, f=0) -> (s? t:f=w496:i32)
                n202 = Select(t=-1, s=w492, f=0) -> (s? t:f=w493:i32)
                n203 = call <vilib>:"WPI_MotorControlSetOutput.vi"("error in (no error)"=w485, "Output"=w496, "MotorControlDevRef"=w486) -> ("MotorControlDevRef"=w472:T1)  [unwired: 6 in, 2 out]
                n204 = call <vilib>:"WPI_MotorControlSetOutput.vi"("error in (no error)"=w481, "Output"=w504, "MotorControlDevRef"=w482) -> ("MotorControlDevRef"=w471:T1)  [unwired: 6 in, 2 out]
                n205 = call <vilib>:"WPI_MotorControlSetOutput.vi"("error in (no error)"=w483, "Output"=w505, "MotorControlDevRef"=w484) -> ("MotorControlDevRef"=w470:T1)  [unwired: 6 in, 2 out]
                n206 = call <vilib>:"WPI_MotorControlSetOutput.vi"("error in (no error)"=w489, "Output"=w493, "MotorControlDevRef"=w490) -> ("MotorControlDevRef"=w469:T1)  [unwired: 6 in, 2 out]
                n207 = Equal?(x=w496, y=0) -> (x = y?=w474:bool)
              }
            }
            frame #4 {
              w523 = 0.0
              n208 = call <vilib>:"WPI_CANTalonSRX_SetSensorPosition.vi"("New Sensor Position"=w523, "CAN Talon SRX Ref"=w522) -> ("CAN Talon SRX Ref"=w521:T1)  [unwired: 8 in, 1 out]
              n209 = call <vilib>:"WPI_CANTalonSRX_SetSensorPosition.vi"("New Sensor Position"=w523, "CAN Talon SRX Ref"=w515) -> ("CAN Talon SRX Ref"=w520:T1)  [unwired: 8 in, 1 out]
              n210 = call <vilib>:"WPI_CANTalonSRX_SetSensorPosition.vi"("New Sensor Position"=w523, "CAN Talon SRX Ref"=w516) -> ("CAN Talon SRX Ref"=w519:T1)  [unwired: 8 in, 1 out]
              n211 = call <vilib>:"WPI_CANTalonSRX_SetSensorPosition.vi"("New Sensor Position"=w523, "CAN Talon SRX Ref"=w517) -> ("CAN Talon SRX Ref"=w518:T1)  [unwired: 8 in, 1 out]
            }
            frame #5 {
              # "Forewards 20 in"
              n212 = while {
                tunnel: w527 -> [w532]
                tunnel: w526 -> [w531]
                tunnel: w525 -> [w530]
                tunnel: w524 -> [w529]
                stop <- w545 stop-if-true
                n213 = call <vilib>:"WPI_CANTalonSRX_GetStatus.vi"("CAN Talon SRX Ref"=w532) -> ("Talon SRX Status"=w541:T5, "CAN Talon SRX Ref"=w540:T1)  [unwired: 8 in, 1 out]
                n214 = call <vilib>:"WPI_CANTalonSRX_GetStatus.vi"("CAN Talon SRX Ref"=w531) -> ("Talon SRX Status"=w544:T5, "CAN Talon SRX Ref"=w537:T1)  [unwired: 8 in, 1 out]
                n215 = call <vilib>:"WPI_CANTalonSRX_GetStatus.vi"("CAN Talon SRX Ref"=w530) -> ("Talon SRX Status"=w543:T5, "CAN Talon SRX Ref"=w539:T1)  [unwired: 8 in, 1 out]
                n216 = call <vilib>:"WPI_CANTalonSRX_GetStatus.vi"("CAN Talon SRX Ref"=w529) -> ("Talon SRX Status"=w542:T5, "CAN Talon SRX Ref"=w538:T1)  [unwired: 8 in, 1 out]
                n217 = Unbundle By Name(w541) -> ("Encoder Position"=w533:dbl)
                n218 = Unbundle By Name(w544) -> ("Encoder Position"=w536:dbl)
                n219 = Unbundle By Name(w543) -> ("Encoder Position"=w534:dbl)
                n220 = Unbundle By Name(w542) -> ("Encoder Position"=w535:dbl)
                n221 = Less?(x=w533, y=20) -> (x < y?=w549:bool)
                n222 = Less?(x=w536, y=20) -> (x < y?=w557:bool)
                n223 = Less?(x=w534, y=20) -> (x < y?=w555:bool)
                n224 = Less?(x=w535, y=20) -> (x < y?=w556:bool)
                n225 = Select(t=1, s=w549, f=0) -> (s? t:f=w546:i32)
                n226 = Select(t=1, s=w557, f=0) -> (s? t:f=w560:i32)
                n227 = Select(t=1, s=w555, f=0) -> (s? t:f=w558:i32)
                n228 = Select(t=1, s=w556, f=0) -> (s? t:f=w559:i32)
                n229 = call <vilib>:"WPI_MotorControlSetOutput.vi"("Output"=w546, "MotorControlDevRef"=w540) -> ()  [unwired: 7 in, 3 out]
                n230 = call <vilib>:"WPI_MotorControlSetOutput.vi"("Output"=w560, "MotorControlDevRef"=w537) -> ()  [unwired: 7 in, 3 out]
                n231 = call <vilib>:"WPI_MotorControlSetOutput.vi"("Output"=w558, "MotorControlDevRef"=w539) -> ()  [unwired: 7 in, 3 out]
                n232 = call <vilib>:"WPI_MotorControlSetOutput.vi"("Output"=w559, "MotorControlDevRef"=w538) -> ()  [unwired: 7 in, 3 out]
                n233 = Equal?(x=w546, y=0) -> (x = y?=w545:bool)
              }
            }
          }
        }
        frame Enabled {
        }
      }
    }
    frame "Left Position" {
      # "Left"
      # "3"
      # "2"
      # "1"
      # "0"
      n234 = call <vilib>:"WPI_MotorControlRefNum Registry Get.vi"("refnum name"="Right Back Motor") -> ("MotorControlDevRef"=w566:T1)  [unwired: 9 in, 1 out]
      n235 = call <vilib>:"WPI_MotorControlRefNum Registry Get.vi"("refnum name"="Left Front Motor") -> ("MotorControlDevRef"=w567:T1)  [unwired: 9 in, 1 out]
      n236 = call <vilib>:"WPI_MotorControlRefNum Registry Get.vi"("refnum name"="Right Front Motor") -> ("MotorControlDevRef"=w568:T1)  [unwired: 9 in, 1 out]
      n237 = call <vilib>:"WPI_MotorControlRefNum Registry Get.vi"("refnum name"="Left Back Motor") -> ("MotorControlDevRef"=w569:T1)  [unwired: 9 in, 1 out]
      n238 = flat-sequence {
        tunnel: [w617] -> w609
        tunnel: [w616] -> w608
        tunnel: [w615] -> w607
        tunnel: [w614] -> w606
        tunnel: w569 -> [w613]
        tunnel: w568 -> [w612]
        tunnel: w567 -> [w611]
        tunnel: w566 -> [w610]
        tunnel: w609 -> [w619]
        tunnel: w608 -> [w620]
        tunnel: w607 -> [w621]
        tunnel: w606 -> [w622]
        tunnel: [w626] -> w573
        tunnel: [w625] -> w572
        tunnel: [w624] -> w571
        tunnel: [w623] -> w570
        tunnel: [w676] -> w605
        tunnel: [w675] -> w604
        tunnel: [w674] -> w603
        tunnel: [w673] -> w602
        tunnel: w573 -> [w672]
        tunnel: w572 -> [w671]
        tunnel: w571 -> [w670]
        tunnel: w570 -> [w669]
        tunnel: w605 -> [w685]
        tunnel: w604 -> [w684]
        tunnel: w603 -> [w683]
        tunnel: w602 -> [w682]
        tunnel: [w681] -> w601
        tunnel: [w680] -> w600
        tunnel: [w679] -> w599
        tunnel: [w678] -> w598
        tunnel: w601 -> [w718]
        tunnel: w600 -> [w717]
        tunnel: w599 -> [w716]
        tunnel: w598 -> [w715]
        tunnel: [w714] -> w597
        tunnel: [w713] -> w596
        tunnel: [w712] -> w595
        tunnel: [w711] -> w594
        tunnel: w597 -> [w724]
        tunnel: w596 -> [w725]
        tunnel: w595 -> [w726]
        tunnel: w594 -> [w727]
        tunnel: [w723] -> w593
        tunnel: [w722] -> w592
        tunnel: [w721] -> w591
        tunnel: [w720] -> w590
        tunnel: w593 -> [w777]
        tunnel: w592 -> [w775]
        tunnel: w591 -> [w773]
        tunnel: w590 -> [w771]
        tunnel: [w776] -> w589
        tunnel: [w774] -> w588
        tunnel: [w772] -> w587
        tunnel: [w770] -> w586
        tunnel: w589 -> [w782]
        tunnel: w588 -> [w781]
        tunnel: w587 -> [w780]
        tunnel: w586 -> [w779]
        tunnel: [w782] -> w585
        tunnel: [w781] -> w584
        tunnel: [w780] -> w583
        tunnel: [w779] -> w582
        tunnel: w585 -> [w797]
        tunnel: w584 -> [w796]
        tunnel: w583 -> [w795]
        tunnel: w582 -> [w794]
        tunnel: [w793] -> w581
        tunnel: [w792] -> w580
        tunnel: [w791] -> w579
        tunnel: [w790] -> w578
        tunnel: w581 -> [w803]
        tunnel: w580 -> [w804]
        tunnel: w579 -> [w805]
        tunnel: w578 -> [w806]
        tunnel: [w802] -> _
        tunnel: [w801] -> _
        tunnel: [w800] -> _
        tunnel: [w799] -> _
        frame #0 {
          w618 = 0.0
          n239 = call <vilib>:"WPI_CANTalonSRX_SetSensorPosition.vi"("New Sensor Position"=w618, "CAN Talon SRX Ref"=w610) -> ("CAN Talon SRX Ref"=w614:T1)  [unwired: 8 in, 1 out]
          n240 = call <vilib>:"WPI_CANTalonSRX_SetSensorPosition.vi"("New Sensor Position"=w618, "CAN Talon SRX Ref"=w611) -> ("CAN Talon SRX Ref"=w615:T1)  [unwired: 8 in, 1 out]
          n241 = call <vilib>:"WPI_CANTalonSRX_SetSensorPosition.vi"("New Sensor Position"=w618, "CAN Talon SRX Ref"=w612) -> ("CAN Talon SRX Ref"=w616:T1)  [unwired: 8 in, 1 out]
          n242 = call <vilib>:"WPI_CANTalonSRX_SetSensorPosition.vi"("New Sensor Position"=w618, "CAN Talon SRX Ref"=w613) -> ("CAN Talon SRX Ref"=w617:T1)  [unwired: 8 in, 1 out]
        }
        frame #1 {
          n243 = while {
            tunnel: [w635] -> w623
            tunnel: [w634] -> w626
            tunnel: [w633] -> w625
            tunnel: [w632] -> w624
            tunnel: w622 -> [w630]
            tunnel: w621 -> [w629]
            tunnel: w620 -> [w628]
            tunnel: w619 -> [w627]
            stop <- w649 stop-if-true
            n244 = call <vilib>:"WPI_CANTalonSRX_GetStatus.vi"("CAN Talon SRX Ref"=w630) -> ("Talon SRX Status"=w645:T5, "CAN Talon SRX Ref"=w644:T1)  [unwired: 8 in, 1 out]
            n245 = call <vilib>:"WPI_CANTalonSRX_GetStatus.vi"("CAN Talon SRX Ref"=w629) -> ("Talon SRX Status"=w648:T5, "CAN Talon SRX Ref"=w641:T1)  [unwired: 8 in, 1 out]
            n246 = call <vilib>:"WPI_CANTalonSRX_GetStatus.vi"("CAN Talon SRX Ref"=w628) -> ("Talon SRX Status"=w647:T5, "CAN Talon SRX Ref"=w643:T1)  [unwired: 8 in, 1 out]
            n247 = call <vilib>:"WPI_CANTalonSRX_GetStatus.vi"("CAN Talon SRX Ref"=w627) -> ("Talon SRX Status"=w646:T5, "CAN Talon SRX Ref"=w642:T1)  [unwired: 8 in, 1 out]
            n248 = Unbundle By Name(w645) -> ("Encoder Position"=w637:dbl)
            n249 = Unbundle By Name(w648) -> ("Encoder Position"=w640:dbl)
            n250 = Unbundle By Name(w647) -> ("Encoder Position"=w638:dbl)
            n251 = Unbundle By Name(w646) -> ("Encoder Position"=w639:dbl)
            n252 = Less?(x=w637, y=20) -> (x < y?=w653:bool)
            n253 = Less?(x=w640, y=20) -> (x < y?=w661:bool)
            n254 = Less?(x=w638, y=20) -> (x < y?=w659:bool)
            n255 = Less?(x=w639, y=20) -> (x < y?=w660:bool)
            n256 = Select(t=1, s=w653, f=0) -> (s? t:f=w650:i32)
            n257 = Select(t=1, s=w661, f=0) -> (s? t:f=w663:i32)
            n258 = Select(t=1, s=w659, f=0) -> (s? t:f=w662:i32)
            n259 = Select(t=1, s=w660, f=0) -> (s? t:f=w631:i32)
            n260 = call <vilib>:"WPI_MotorControlSetOutput.vi"("Output"=w650, "MotorControlDevRef"=w644) -> ("MotorControlDevRef"=w635:T1)  [unwired: 7 in, 2 out]
            n261 = call <vilib>:"WPI_MotorControlSetOutput.vi"("Output"=w663, "MotorControlDevRef"=w641) -> ("MotorControlDevRef"=w632:T1)  [unwired: 7 in, 2 out]
            n262 = call <vilib>:"WPI_MotorControlSetOutput.vi"("Output"=w662, "MotorControlDevRef"=w643) -> ("MotorControlDevRef"=w633:T1)  [unwired: 7 in, 2 out]
            n263 = call <vilib>:"WPI_MotorControlSetOutput.vi"("Output"=w631, "MotorControlDevRef"=w642) -> ("MotorControlDevRef"=w634:T1)  [unwired: 7 in, 2 out]
            n264 = Equal?(x=w631, y=0) -> (x = y?=w649:bool)
          }
        }
        frame #2 {
          w677 = 0.0
          n265 = call <vilib>:"WPI_CANTalonSRX_SetSensorPosition.vi"("New Sensor Position"=w677, "CAN Talon SRX Ref"=w669) -> ("CAN Talon SRX Ref"=w676:T1)  [unwired: 8 in, 1 out]
          n266 = call <vilib>:"WPI_CANTalonSRX_SetSensorPosition.vi"("New Sensor Position"=w677, "CAN Talon SRX Ref"=w670) -> ("CAN Talon SRX Ref"=w675:T1)  [unwired: 8 in, 1 out]
          n267 = call <vilib>:"WPI_CANTalonSRX_SetSensorPosition.vi"("New Sensor Position"=w677, "CAN Talon SRX Ref"=w671) -> ("CAN Talon SRX Ref"=w674:T1)  [unwired: 8 in, 1 out]
          n268 = call <vilib>:"WPI_CANTalonSRX_SetSensorPosition.vi"("New Sensor Position"=w677, "CAN Talon SRX Ref"=w672) -> ("CAN Talon SRX Ref"=w673:T1)  [unwired: 8 in, 1 out]
        }
        frame #3 {
          n269 = while {
            tunnel: w685 -> [w699]
            tunnel: w684 -> [w698]
            tunnel: w683 -> [w697]
            tunnel: w682 -> [w696]
            tunnel: [w695] -> w681
            tunnel: [w694] -> w680
            tunnel: [w693] -> w679
            tunnel: [w692] -> w678
            stop <- w688 stop-if-true
            w701 = 100
            # "vision"
            n270 = Wait (ms)(milliseconds to wait=w701) -> (millisecond timer value=w702:u32)
            n271 = Equal?(x=w702, y=w701) -> (x = y?=w700:bool)
            n272 = case shown="True" w700 {
              tunnel: [0 w707] -> w691
              tunnel: [TRUE w706] -> w687
              frame False {
              }
              frame True {
                # "distance is far"
                n273 = global read "Robot Global Data.vi" "Distance"() -> (w705:dbl)
                n274 = Greater?(x=w705, y=1) -> (0:w706:bool)
                n275 = Select(t=1, s=w706, f=0) -> (s? t:f=w707:i32)
              }
            }
            n276 = Negate(x=w691) -> (-x=w690:i32)
            n277 = Negate(x=w691) -> (-x=w689:i32)
            n278 = call <vilib>:"WPI_MotorControlSetOutput.vi"("Output"=w690, "MotorControlDevRef"=w699) -> ("MotorControlDevRef"=w695:T1)  [unwired: 7 in, 2 out]
            n279 = call <vilib>:"WPI_MotorControlSetOutput.vi"("Output"=w689, "MotorControlDevRef"=w698) -> ("MotorControlDevRef"=w694:T1)  [unwired: 7 in, 2 out]
            n280 = call <vilib>:"WPI_MotorControlSetOutput.vi"("Output"=w691, "MotorControlDevRef"=w697) -> ("MotorControlDevRef"=w693:T1)  [unwired: 7 in, 2 out]
            n281 = call <vilib>:"WPI_MotorControlSetOutput.vi"("Output"=w691, "MotorControlDevRef"=w696) -> ("MotorControlDevRef"=w692:T1)  [unwired: 7 in, 2 out]
            n282 = And(x=w687, y=FALSE) -> (x .and. y?=w688:bool)
          }
        }
        frame #4 {
          w719 = 0.0
          n283 = call <vilib>:"WPI_CANTalonSRX_SetSensorPosition.vi"("New Sensor Position"=w719, "CAN Talon SRX Ref"=w718) -> ("CAN Talon SRX Ref"=w711:T1)  [unwired: 8 in, 1 out]
          n284 = call <vilib>:"WPI_CANTalonSRX_SetSensorPosition.vi"("New Sensor Position"=w719, "CAN Talon SRX Ref"=w717) -> ("CAN Talon SRX Ref"=w712:T1)  [unwired: 8 in, 1 out]
          n285 = call <vilib>:"WPI_CANTalonSRX_SetSensorPosition.vi"("New Sensor Position"=w719, "CAN Talon SRX Ref"=w716) -> ("CAN Talon SRX Ref"=w713:T1)  [unwired: 8 in, 1 out]
          n286 = call <vilib>:"WPI_CANTalonSRX_SetSensorPosition.vi"("New Sensor Position"=w719, "CAN Talon SRX Ref"=w715) -> ("CAN Talon SRX Ref"=w714:T1)  [unwired: 8 in, 1 out]
        }
        frame #5 {
          n287 = while {
            tunnel: w727 -> [w737]
            tunnel: w726 -> [w736]
            tunnel: w725 -> [w735]
            tunnel: w724 -> [w734]
            tunnel: [w732] -> w723
            tunnel: [w731] -> w720
            tunnel: [w730] -> w721
            tunnel: [w729] -> w722
            stop <- w750 stop-if-true
            n288 = call <vilib>:"WPI_CANTalonSRX_GetStatus.vi"("CAN Talon SRX Ref"=w737) -> ("Talon SRX Status"=w746:T5, "CAN Talon SRX Ref"=w745:T1)  [unwired: 8 in, 1 out]
            n289 = call <vilib>:"WPI_CANTalonSRX_GetStatus.vi"("CAN Talon SRX Ref"=w736) -> ("Talon SRX Status"=w749:T5, "CAN Talon SRX Ref"=w742:T1)  [unwired: 8 in, 1 out]
            n290 = call <vilib>:"WPI_CANTalonSRX_GetStatus.vi"("CAN Talon SRX Ref"=w735) -> ("Talon SRX Status"=w748:T5, "CAN Talon SRX Ref"=w744:T1)  [unwired: 8 in, 1 out]
            n291 = call <vilib>:"WPI_CANTalonSRX_GetStatus.vi"("CAN Talon SRX Ref"=w734) -> ("Talon SRX Status"=w747:T5, "CAN Talon SRX Ref"=w743:T1)  [unwired: 8 in, 1 out]
            n292 = Unbundle By Name(w746) -> ("Encoder Position"=w738:dbl)
            n293 = Unbundle By Name(w749) -> ("Encoder Position"=w741:dbl)
            n294 = Unbundle By Name(w748) -> ("Encoder Position"=w739:dbl)
            n295 = Unbundle By Name(w747) -> ("Encoder Position"=w740:dbl)
            n296 = Greater?(x=w738, y=-5) -> (0:w754:bool)
            n297 = Greater?(x=w741, y=-5) -> (0:w762:bool)
            n298 = Less?(x=w739, y=5) -> (x < y?=w760:bool)
            n299 = Less?(x=w740, y=5) -> (x < y?=w761:bool)
            n300 = Select(t=-1, s=w754, f=0) -> (s? t:f=w751:i32)
            n301 = Select(t=-1, s=w762, f=0) -> (s? t:f=w764:i32)
            n302 = Select(t=1, s=w760, f=0) -> (s? t:f=w763:i32)
            n303 = Select(t=1, s=w761, f=0) -> (s? t:f=w728:i32)
            n304 = call <vilib>:"WPI_MotorControlSetOutput.vi"("Output"=w751, "MotorControlDevRef"=w745) -> ("MotorControlDevRef"=w732:T1)  [unwired: 7 in, 2 out]
            n305 = call <vilib>:"WPI_MotorControlSetOutput.vi"("Output"=w764, "MotorControlDevRef"=w742) -> ("MotorControlDevRef"=w729:T1)  [unwired: 7 in, 2 out]
            n306 = call <vilib>:"WPI_MotorControlSetOutput.vi"("Output"=w763, "MotorControlDevRef"=w744) -> ("MotorControlDevRef"=w730:T1)  [unwired: 7 in, 2 out]
            n307 = call <vilib>:"WPI_MotorControlSetOutput.vi"("Output"=w728, "MotorControlDevRef"=w743) -> ("MotorControlDevRef"=w731:T1)  [unwired: 7 in, 2 out]
            n308 = Equal?(x=w728, y=0) -> (x = y?=w750:bool)
          }
        }
        frame #6 {
          w778 = 0.0
          n309 = call <vilib>:"WPI_CANTalonSRX_SetSensorPosition.vi"("New Sensor Position"=w778, "CAN Talon SRX Ref"=w777) -> ("CAN Talon SRX Ref"=w776:T1)  [unwired: 8 in, 1 out]
          n310 = call <vilib>:"WPI_CANTalonSRX_SetSensorPosition.vi"("New Sensor Position"=w778, "CAN Talon SRX Ref"=w775) -> ("CAN Talon SRX Ref"=w774:T1)  [unwired: 8 in, 1 out]
          n311 = call <vilib>:"WPI_CANTalonSRX_SetSensorPosition.vi"("New Sensor Position"=w778, "CAN Talon SRX Ref"=w773) -> ("CAN Talon SRX Ref"=w772:T1)  [unwired: 8 in, 1 out]
          n312 = call <vilib>:"WPI_CANTalonSRX_SetSensorPosition.vi"("New Sensor Position"=w778, "CAN Talon SRX Ref"=w771) -> ("CAN Talon SRX Ref"=w770:T1)  [unwired: 8 in, 1 out]
        }
        frame #7 {
          n313 = while {
            stop <- w783 stop-if-true
            w784 = 1000
            n314 = call <vilib>:"WPI_MotorControlRefNum Registry Get.vi"("refnum name"="Gear Arm") -> ("error out"=w789:errorcluster, "MotorControlDevRef"=w788:T1)  [unwired: 9 in]
            n315 = Wait (ms)(milliseconds to wait=w784) -> (millisecond timer value=w785:u32)
            n316 = call <vilib>:"WPI_MotorControlSetOutput.vi"("error in (no error)"=w789, "Output"=-1, "MotorControlDevRef"=w788) -> ()  [unwired: 6 in, 3 out]
            n317 = Equal?(x=w785, y=w784) -> (x = y?=w783:bool)
          }
        }
        frame #8 {
          w798 = 0.0
          n318 = call <vilib>:"WPI_CANTalonSRX_SetSensorPosition.vi"("New Sensor Position"=w798, "CAN Talon SRX Ref"=w797) -> ("CAN Talon SRX Ref"=w790:T1)  [unwired: 8 in, 1 out]
          n319 = call <vilib>:"WPI_CANTalonSRX_SetSensorPosition.vi"("New Sensor Position"=w798, "CAN Talon SRX Ref"=w796) -> ("CAN Talon SRX Ref"=w791:T1)  [unwired: 8 in, 1 out]
          n320 = call <vilib>:"WPI_CANTalonSRX_SetSensorPosition.vi"("New Sensor Position"=w798, "CAN Talon SRX Ref"=w795) -> ("CAN Talon SRX Ref"=w792:T1)  [unwired: 8 in, 1 out]
          n321 = call <vilib>:"WPI_CANTalonSRX_SetSensorPosition.vi"("New Sensor Position"=w798, "CAN Talon SRX Ref"=w794) -> ("CAN Talon SRX Ref"=w793:T1)  [unwired: 8 in, 1 out]
        }
        frame #9 {
          n322 = while {
            tunnel: w806 -> [w816]
            tunnel: w805 -> [w815]
            tunnel: w804 -> [w814]
            tunnel: w803 -> [w813]
            tunnel: [w811] -> w802
            tunnel: [w810] -> w799
            tunnel: [w809] -> w800
            tunnel: [w808] -> w801
            stop <- w829 stop-if-true
            n323 = call <vilib>:"WPI_CANTalonSRX_GetStatus.vi"("CAN Talon SRX Ref"=w816) -> ("Talon SRX Status"=w825:T5, "CAN Talon SRX Ref"=w824:T1)  [unwired: 8 in, 1 out]
            n324 = call <vilib>:"WPI_CANTalonSRX_GetStatus.vi"("CAN Talon SRX Ref"=w815) -> ("Talon SRX Status"=w828:T5, "CAN Talon SRX Ref"=w821:T1)  [unwired: 8 in, 1 out]
            n325 = call <vilib>:"WPI_CANTalonSRX_GetStatus.vi"("CAN Talon SRX Ref"=w814) -> ("Talon SRX Status"=w827:T5, "CAN Talon SRX Ref"=w823:T1)  [unwired: 8 in, 1 out]
            n326 = call <vilib>:"WPI_CANTalonSRX_GetStatus.vi"("CAN Talon SRX Ref"=w813) -> ("Talon SRX Status"=w826:T5, "CAN Talon SRX Ref"=w822:T1)  [unwired: 8 in, 1 out]
            n327 = Unbundle By Name(w825) -> ("Encoder Position"=w817:dbl)
            n328 = Unbundle By Name(w828) -> ("Encoder Position"=w820:dbl)
            n329 = Unbundle By Name(w827) -> ("Encoder Position"=w818:dbl)
            n330 = Unbundle By Name(w826) -> ("Encoder Position"=w819:dbl)
            n331 = Less?(x=w817, y=5) -> (x < y?=w833:bool)
            n332 = Less?(x=w820, y=5) -> (x < y?=w841:bool)
            n333 = Greater?(x=w818, y=-5) -> (0:w839:bool)
            n334 = Greater?(x=w819, y=-5) -> (0:w840:bool)
            n335 = Select(t=1, s=w833, f=0) -> (s? t:f=w830:i32)
            n336 = Select(t=1, s=w841, f=0) -> (s? t:f=w843:i32)
            n337 = Select(t=-1, s=w839, f=0) -> (s? t:f=w842:i32)
            n338 = Select(t=-1, s=w840, f=0) -> (s? t:f=w807:i32)
            n339 = call <vilib>:"WPI_MotorControlSetOutput.vi"("Output"=w830, "MotorControlDevRef"=w824) -> ("MotorControlDevRef"=w811:T1)  [unwired: 7 in, 2 out]
            n340 = call <vilib>:"WPI_MotorControlSetOutput.vi"("Output"=w843, "MotorControlDevRef"=w821) -> ("MotorControlDevRef"=w808:T1)  [unwired: 7 in, 2 out]
            n341 = call <vilib>:"WPI_MotorControlSetOutput.vi"("Output"=w842, "MotorControlDevRef"=w823) -> ("MotorControlDevRef"=w809:T1)  [unwired: 7 in, 2 out]
            n342 = call <vilib>:"WPI_MotorControlSetOutput.vi"("Output"=w807, "MotorControlDevRef"=w822) -> ("MotorControlDevRef"=w810:T1)  [unwired: 7 in, 2 out]
            n343 = Equal?(x=w807, y=0) -> (x = y?=w829:bool)
          }
        }
      }
    }
    frame Default {
      # "Right"
      # "3"
      # "2"
      # "1"
      # "0"
      # "foreward 20 in"
      n344 = call <vilib>:"WPI_MotorControlRefNum Registry Get.vi"("refnum name"="Right Back Motor") -> ("MotorControlDevRef"=w856:T1)  [unwired: 9 in, 1 out]
      n345 = call <vilib>:"WPI_MotorControlRefNum Registry Get.vi"("refnum name"="Left Front Motor") -> ("MotorControlDevRef"=w855:T1)  [unwired: 9 in, 1 out]
      n346 = call <vilib>:"WPI_MotorControlRefNum Registry Get.vi"("refnum name"="Right Front Motor") -> ("MotorControlDevRef"=w854:T1)  [unwired: 9 in, 1 out]
      n347 = call <vilib>:"WPI_MotorControlRefNum Registry Get.vi"("refnum name"="Left Back Motor") -> ("MotorControlDevRef"=w853:T1)  [unwired: 9 in, 1 out]
      n348 = flat-sequence {
        tunnel: w856 -> [w868]
        tunnel: w855 -> [w867]
        tunnel: w854 -> [w866]
        tunnel: w853 -> [w865]
        tunnel: [w864] -> w852
        tunnel: [w863] -> w851
        tunnel: [w862] -> w850
        tunnel: [w861] -> w849
        tunnel: w852 -> [w873]
        tunnel: w851 -> [w872]
        tunnel: w850 -> [w871]
        tunnel: w849 -> [w870]
        frame #0 {
          w869 = 0.0
          n349 = call <vilib>:"WPI_CANTalonSRX_SetSensorPosition.vi"("New Sensor Position"=w869, "CAN Talon SRX Ref"=w868) -> ("CAN Talon SRX Ref"=w861:T1)  [unwired: 8 in, 1 out]
          n350 = call <vilib>:"WPI_CANTalonSRX_SetSensorPosition.vi"("New Sensor Position"=w869, "CAN Talon SRX Ref"=w867) -> ("CAN Talon SRX Ref"=w862:T1)  [unwired: 8 in, 1 out]
          n351 = call <vilib>:"WPI_CANTalonSRX_SetSensorPosition.vi"("New Sensor Position"=w869, "CAN Talon SRX Ref"=w866) -> ("CAN Talon SRX Ref"=w863:T1)  [unwired: 8 in, 1 out]
          n352 = call <vilib>:"WPI_CANTalonSRX_SetSensorPosition.vi"("New Sensor Position"=w869, "CAN Talon SRX Ref"=w865) -> ("CAN Talon SRX Ref"=w864:T1)  [unwired: 8 in, 1 out]
        }
        frame #1 {
          n353 = while {
            tunnel: [w886] -> _
            tunnel: [w885] -> _
            tunnel: [w884] -> _
            tunnel: [w883] -> _
            tunnel: w873 -> [w877]
            tunnel: w872 -> [w876]
            tunnel: w871 -> [w875]
            tunnel: w870 -> [w874]
            stop <- w878 stop-if-true
            n354 = call <vilib>:"WPI_CANTalonSRX_GetStatus.vi"("CAN Talon SRX Ref"=w874) -> ("Talon SRX Status"=w896:T5, "CAN Talon SRX Ref"=w895:T1)  [unwired: 8 in, 1 out]
            n355 = call <vilib>:"WPI_CANTalonSRX_GetStatus.vi"("CAN Talon SRX Ref"=w875) -> ("Talon SRX Status"=w899:T5, "CAN Talon SRX Ref"=w892:T1)  [unwired: 8 in, 1 out]
            n356 = call <vilib>:"WPI_CANTalonSRX_GetStatus.vi"("CAN Talon SRX Ref"=w876) -> ("Talon SRX Status"=w898:T5, "CAN Talon SRX Ref"=w894:T1)  [unwired: 8 in, 1 out]
            n357 = call <vilib>:"WPI_CANTalonSRX_GetStatus.vi"("CAN Talon SRX Ref"=w877) -> ("Talon SRX Status"=w897:T5, "CAN Talon SRX Ref"=w893:T1)  [unwired: 8 in, 1 out]
            n358 = Unbundle By Name(w896) -> ("Encoder Position"=w888:dbl)
            n359 = Unbundle By Name(w899) -> ("Encoder Position"=w891:dbl)
            n360 = Unbundle By Name(w898) -> ("Encoder Position"=w889:dbl)
            n361 = Unbundle By Name(w897) -> ("Encoder Position"=w890:dbl)
            n362 = Less?(x=w888, y=20) -> (x < y?=w902:bool)
            n363 = Less?(x=w891, y=20) -> (x < y?=w910:bool)
            n364 = Less?(x=w889, y=20) -> (x < y?=w908:bool)
            n365 = Less?(x=w890, y=20) -> (x < y?=w909:bool)
            n366 = Select(t=1, s=w902, f=0) -> (s? t:f=w900:i32)
            n367 = Select(t=1, s=w910, f=0) -> (s? t:f=w911:i32)
            n368 = Select(t=1, s=w908, f=0) -> (s? t:f=w882:i32)
            n369 = Select(t=1, s=w909, f=0) -> (s? t:f=w881:i32)
            n370 = call <vilib>:"WPI_MotorControlSetOutput.vi"("Output"=w900, "MotorControlDevRef"=w895) -> ("MotorControlDevRef"=w886:T1)  [unwired: 7 in, 2 out]
            n371 = call <vilib>:"WPI_MotorControlSetOutput.vi"("Output"=w911, "MotorControlDevRef"=w892) -> ("MotorControlDevRef"=w883:T1)  [unwired: 7 in, 2 out]
            n372 = call <vilib>:"WPI_MotorControlSetOutput.vi"("Output"=w882, "MotorControlDevRef"=w894) -> ("MotorControlDevRef"=w884:T1)  [unwired: 7 in, 2 out]
            n373 = call <vilib>:"WPI_MotorControlSetOutput.vi"("Output"=w881, "MotorControlDevRef"=w893) -> ("MotorControlDevRef"=w885:T1)  [unwired: 7 in, 2 out]
            n374 = Equal To 0?(x=w882) -> (x = 0?=w880:bool)
            n375 = Equal To 0?(x=w881) -> (x = 0?=w879:bool)
            n376 = And(x=w880, y=w879) -> (x .and. y?=w878:bool)
          }
        }
      }
    }
  }
